vi "response message.vi"(8 "error in":errorcluster, 11 "params (formatted)":string) -> (0 "error out":errorcluster, 2 "length":i32, 3 "response":string)   [LabVIEW 2014]
doc: "Formats an XML-RPC data type into a message body for inclusion in a response message"
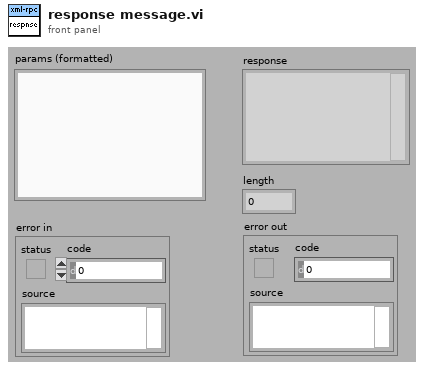
[diagram p1: front panel]
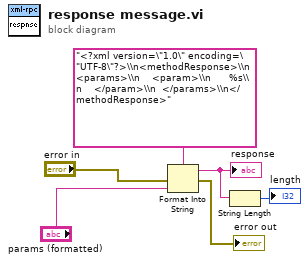
[diagram p0: block diagram]
diagram:
  n1 = Format Into String(format string="<?xml version=\"1.0\" encoding=\"UTF-8\"?>\\n<methodResponse>\\n  <params>\\n    <param>\\n      %s\\n    </param>\\n  </params>\\n</methodResponse>", error in="error in", "params (formatted)") -> (resulting string=w2:string, error out=→"error out":errorcluster)  [unwired: 1 in]
  "response" <- w2
  n2 = String Length(string=w2) -> (length=→"length":i32)
